vi "HarvRoller.vi"(8 "HarvRollerBDesSpd":dbl, 9 "HarvRollerFDesSpd":dbl, 10 "HarvOutElev":dbl, 11 "HarvSetElev":i32) -> (1 "HarvOutRollerB":dbl, 2 "HarvOutRollerF":dbl, 3 "HarvShootEnable":bool)   [LabVIEW 2012]
panel:
  out "HarvOutElev":dbl
  in  "HarvSetElev":i32
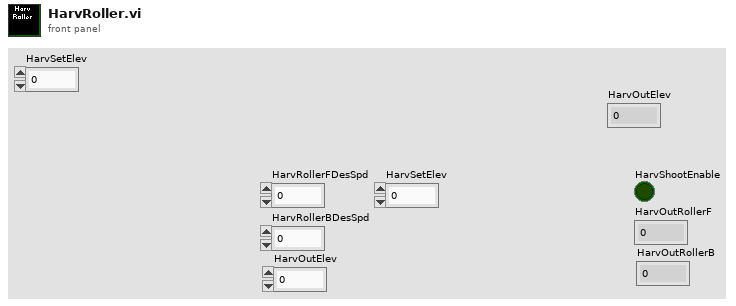
[diagram p1: front panel]
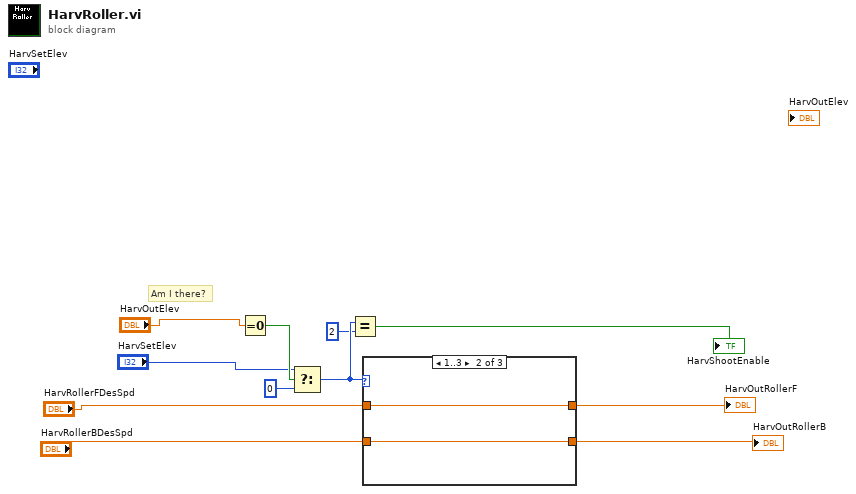
[diagram p0: block diagram]
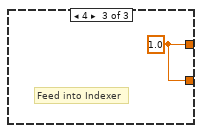
[diagram p3: hidden frame]
diagram:
  # "Am I there?"
  n1 = Equal To 0?(x="HarvOutElev") -> (x = 0?=w9:bool)
  n2 = Select(t="HarvSetElev", s=w9, f=0) -> (s? t:f=w7:i32)
  n3 = Equal?(x=w7, y=2) -> (x = y?=→"HarvShootEnable":bool)
  n4 = case shown="1..3" w7 {
    tunnel: [w13 w15 w16] -> w10
    tunnel: [w12 w14 w16] -> w5
    tunnel: "HarvRollerFDesSpd" -> [w13 w15 _]
    tunnel: "HarvRollerBDesSpd" -> [w12 w14 _]
    frame 0, Default {
      # "DO NOTHING"
    }
    frame 1..3 {
    }
    frame 4 {
      w16 = 1.0 ("HarvRollerFDesSpd")
      # "Feed into Indexer"
    }
  }
  "HarvOutRollerF" <- w10
  "HarvOutRollerB" <- w5
